vi "Root Directory.vi"() -> (2 "root directory":path)   [LabVIEW 2017]
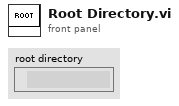
[diagram p1: front panel]
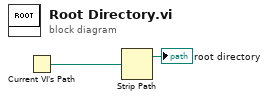
[diagram p0: block diagram]
diagram:
  n1 = Current VI's Path() -> (path=w2:path)
  n2 = Strip Path(path=w2) -> (stripped path=→"root directory":path)  [unwired: 1 out]
